vi "LED Lights Open.vi"(8 "error in":errorcluster, 11 "I2C Bus":T3=enum."Invalid") -> (0 "error out":errorcluster, 3 "output cluster":T1={"I2CDevRef"={"DevStatus"={"status"=FALSE, "code"=0, "source"=""}, "Device Address"=0, "Handle"=0, "I2C Bus"=enum."Invalid"}} {"I2CDevRef"."Device Address" format="%.0x"})   [LabVIEW 2015]
uses:
  <vilib>/Rock Robotics/SystemInterfaces/i2clib/i2c_bus.ctl
  LED Lights Ref.ctl
  <vilib>/Rock Robotics/WPI/I2C/WPI_I2CDevRef.ctl
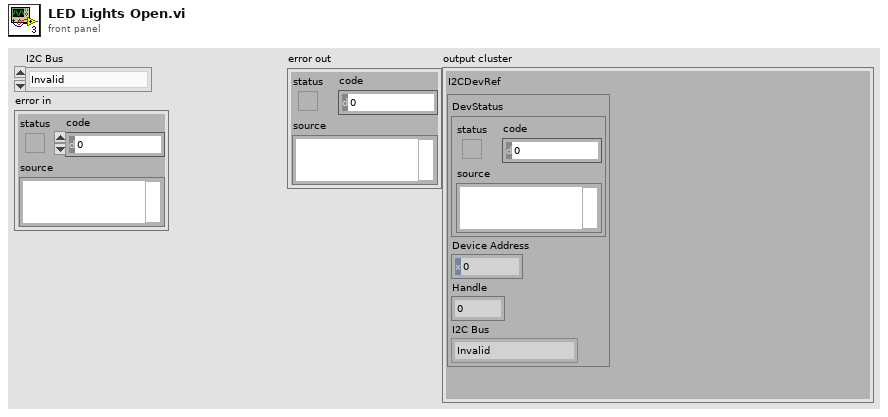
[diagram p1: front panel]
types:
  T1 = typedef "LED Lights Ref.ctl" = cluster{"I2CDevRef":T2}
  T2 = typedef "WPI_I2CDevRef.ctl" = cluster{"DevStatus":errorcluster, "Device Address":u8, "Handle":i32, "I2C Bus":T3}
  T3 = typedef "i2c_bus.ctl" = enum16{"I2C On-Board", "I2C MXP", "Invalid"}
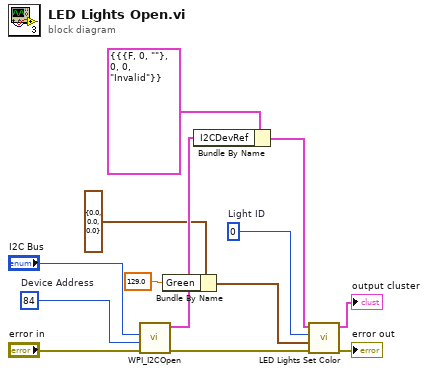
[diagram p0: block diagram]
diagram:
  w3 = u8 0  # Light ID
  w11 = u8 84  # Device Address
  n1 = call <vilib>:"WPI_I2COpen.vi"("error in"="error in", "Device Address"=w11, "I2C Bus"="I2C Bus") -> ("error out"=w1:errorcluster, "I2CDevRef"=w9:T2)  [unwired: 7 in]
  n2 = Bundle By Name(cluster=cluster{"Red":dbl, "Green":dbl, "Blue":dbl} {"Red"=0.0, "Green"=0.0, "Blue"=0.0} ("Color"), "Green"=129.0) -> (w2:cluster{"Red":dbl, "Green":dbl, "Blue":dbl})
  n3 = Bundle By Name(cluster=T1 {"I2CDevRef"={"DevStatus"={"status"=FALSE, "code"=0, "source"=""}, "Device Address"=0, "Handle"=0, "I2C Bus"=enum."Invalid"}} ("LED Lights Ref"), "I2CDevRef"=w9) -> (w4:T1)
  n4 = call "LED Lights Set Color.vi"("error in"=w1, "Color"=w2, "Light ID"=w3, "LED Lights Ref In"=w4) -> ("error out"=→"error out":errorcluster, "LED Lights Ref Out"=→"output cluster":T1)  [unwired: 6 in]
